vi "measure2.vi"() -> ()   [LabVIEW 2018]
doc: "To remove low frequency noise from a measurement, set the aperture to 1/f, where f is a multiple of the noise frequency. Averaging multiple measurements together can further improve the resolution. This example acquires multiple DC voltage measurements. After specifying the instrument descriptor, select the function and range. Specify the aperture time in seconds and set the number of measurements to average. The specified number of measurements are returned, as well as a calculated resolution of the measurements. Auto Zero must be On when averaging."
uses:
  <instrlib>/niDMM/nidmm.llb/niDMM Function.ctl
  <instrlib>/niDMM/nidmm.llb/niDMM Auto Zero.ctl
  <vilib>/Utility/error.llb/DialogType.ctl
  <instrlib>/niDMM/nidmm.llb/niDMM Configure Measurement Digits.vi
panel:
  in  "Timeout (ms)":i32=20000
  out "Effective Number of Digits":dbl format="%.2f"
  out "Waveform Graph":dbl[](graph)
  in  "Sample Count":i32=10
  in  "Auto Zero":T1=1 items=["Auto"=-1, "Off"=0, "On"=1, "Once"=2]
  in  "Measurement Type":T2
  in  "Number of Averages":i32=8
  in  "Aperture time (s)":dbl=0.1 format="%.2p"
  in  "Device Name":refnum<k15>="Dev1"
  in  "Range (Volts)":dbl=10.0 format="%.2p"
  # "For instructions select File >> VI Properties >> Documentation"
  # "Configuration"
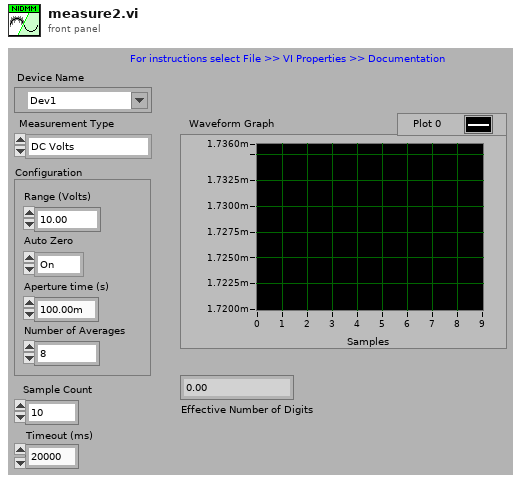
[diagram p1: front panel]
types:
  T1 = typedef "niDMM Auto Zero.ctl" = i32
  T2 = typedef "niDMM Function.ctl" = enum16{"DC Volts", "AC Volts", "DC Current", "AC Current", "2-wire Resistance", "4-wire Resistance", "Diode", "Frequency", "Period", "AC Volts DC Coupled", "Capacitance", "Inductance", "Temperature"}
  T3 = typedef "DialogType.ctl" = u16
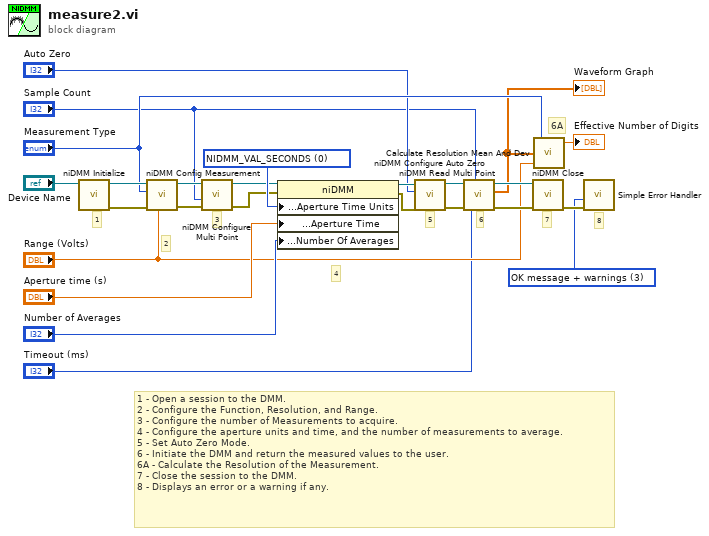
[diagram p0: block diagram]
diagram:
  w1 = T3 3 items=["no dialog", "OK message", "continue or stop message", "OK message + warnings", "continue/stop + warnings"] ("type of dialog (OK msg:1)")
  w22 = 0 items=["NIDMM_VAL_SECONDS", "NIDMM_VAL_POWER_LINE_CYCLES"] ("Configuration Information:Aperture Time Units")
  # "7"
  # "3"
  # "8"
  # "6A"
  # "6"
  # "1 - Open a session to the DMM.\n2 - Configure the Function, Resolution, and Range.\n3 - Configure the number of Measurements to acquire.\n4 - Configure the aperture units and time, and the number of measurements to average.\n5 - Set Auto Zero Mode.\n6 - Initiate the DMM and return the measured values to the user.\n6A - Calculate the Resolution of the Measurement.\n7 - Close the session to the DMM.\n8 - Displays an error or a warning if any."
  # "1"
  # "5"
  # "4"
  # "2"
  n1 = call <instrlib>:"niDMM Initialize.vi"("Instrument Descriptor"="Device Name") -> ("error out"=w24:errorcluster, "instrument handle out"=w25:refnum<k15>)  [unwired: 9 in]
  n2 = call-poly <instrlib>:"niDMM Config Measurement.vi"("Range"="Range (Volts)", "error in (no error)"=w24, "Function"="Measurement Type", "instrument handle"=w25) -> ("error out"=w12:errorcluster, "instrument handle out"=w13:refnum<k15>)  [unwired: 6 in]
  n3 = call <instrlib>:"niDMM Configure Multi Point.vi"("error in (no error)"=w12, "Sample Count"="Sample Count", "instrument handle"=w13) -> ("error out"=w10:errorcluster, "instrument handle out"=w11:refnum<k15>)  [unwired: 7 in]
  n4 = property class="niDMM"(reference=w11, error in=w10, "Configuration:Advanced:Aperture Time Units"=w22, "Configuration:Advanced:Aperture Time"="Aperture time (s)", "Configuration:Advanced:Number Of Averages"="Number of Averages") -> (reference out=w20:refnum<k15>, error out=w19:errorcluster)
  n5 = call <instrlib>:"niDMM Configure Auto Zero.vi"("error in (no error)"=w19, "Auto Zero"="Auto Zero", "instrument handle"=w20) -> ("error out"=w17:errorcluster, "instrument handle out"=w18:refnum<k15>)  [unwired: 7 in]
  n6 = call <instrlib>:"niDMM Read Multi Point.vi"("Maximum Time (msec)"="Timeout (ms)", "Number to Read"="Sample Count", "error in (no error)"=w17, "instrument handle"=w18) -> ("error out"=w8:errorcluster, "Measurements"=w6:dbl[], "instrument handle out"=w9:refnum<k15>)  [unwired: 4 in, 1 out]
  "Waveform Graph" <- w6
  n7 = call <instrlib>:"niDMM Close.vi"("error in (no error)"=w8, "instrument handle"=w9) -> ("error out"=w3:errorcluster)  [unwired: 9 in]
  n8 = call "Calculate Resolution Mean And Dev.vi"("Range"="Range (Volts)", "Array"=w6, "Measurement Type"="Measurement Type") -> ("Resolution"=→"Effective Number of Digits":dbl)  [unwired: 2 out]
  n9 = call <vilib>:"Simple Error Handler.vi"("type of dialog (OK msg:1)"=w1, "error in (no error)"=w3) -> ()  [unwired: 3 in, 5 out]
